vi "item selection type.vi"(11 "Loop data":T2) -> (1 "Type":T1, 3 "Loop data":T2)   [LabVIEW 2020, in "UI_ItemSelect_OpenSource.lvlib"]
uses:
  UI_ItemSelect_OpenSource.lvlib
  Tree item select loop data.ctl
  Item select ref type.ctl
  Tree item loop data.ctl
  Tree item selection indices.ctl
  checkbox state.ctl
  item select tree lock states.ctl
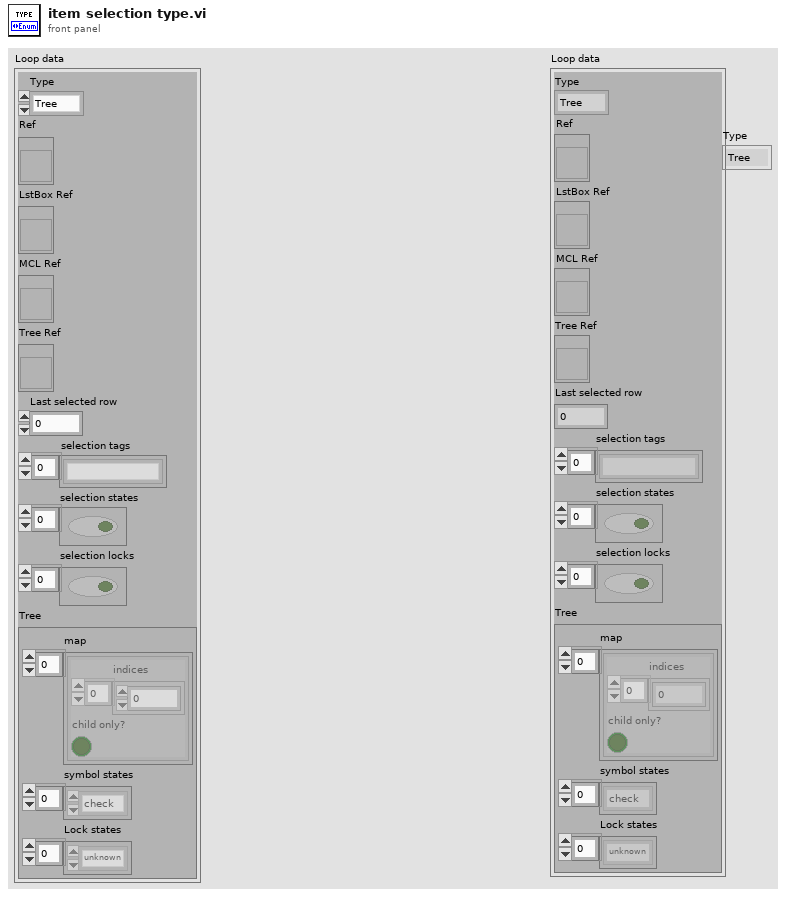
[diagram p1: front panel]
types:
  T1 = typedef "UI_ItemSelect_OpenSource.lvlib/Item select ref type.ctl" = enum16{"Tree", "MCL", "ListBox"}
  T2 = typedef "UI_ItemSelect_OpenSource.lvlib/Tree item select loop data.ctl" = cluster{"Type":T1, "Ref":refnum<vi>, "LstBox Ref":refnum<vi>, "MCL Ref":refnum<vi>, "Tree Ref":refnum<vi>, "Last selected row":i32, "selection tags":string[], "selection states":bool[], "selection locks":bool[], "Tree":T3}
  T3 = typedef "UI_ItemSelect_OpenSource.lvlib/Tree item loop data.ctl" = cluster{"map":T4[], "symbol states":T5[], "Lock states":T6[]}
  T4 = typedef "UI_ItemSelect_OpenSource.lvlib/Tree item selection indices.ctl" = cluster{"indices":i32[], "child only?":bool}
  T5 = typedef "UI_ItemSelect_OpenSource.lvlib/checkbox state.ctl" = enum16{"unknown", "check", "some", "no check"}
  T6 = typedef "UI_ItemSelect_OpenSource.lvlib/item select tree lock states.ctl" = enum16{"unknown", "locked", "unlocked"}
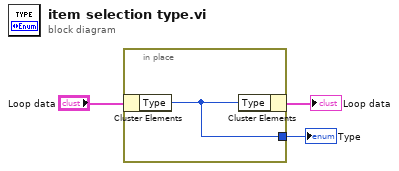
[diagram p0: block diagram]
diagram:
  n1 = in-place {
    in-place-border: [w4] -> w1
    n2 = in-place-cluster #1("Loop data") -> ("Type"=w4:T1)
    n3 = in-place-cluster #1("Type"=w4) -> (→"Loop data":T2)
  }
  "Type" <- w1
